vi "_Clear Capabilities.vi"(8 "error in (no error)":errorcluster, 11 "NodeDiscovery in":refnum<class "DiscoveryService.lvclass">) -> (0 "error out":errorcluster, 3 "NodeDiscovery out":refnum<class "DiscoveryService.lvclass">)   [LabVIEW 2020, in "Vecto.lvlib" / "DiscoveryService.lvclass"]
uses:
  DiscoveryService.lvclass
  DiscoveryService.lvclass/DiscoveryService.ctl
  Node Config/Node Config.lvclass
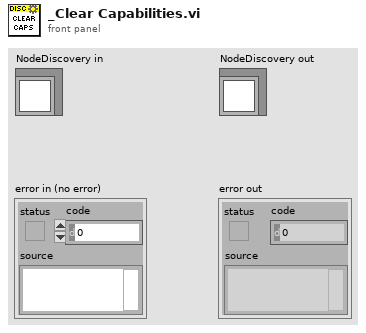
[diagram p1: front panel]
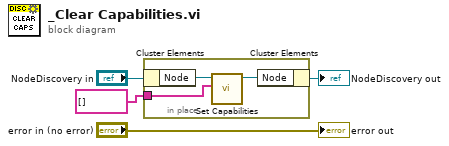
[diagram p0: block diagram]
diagram:
  n1 = in-place {
    in-place-border: string[] [] ("Capabilities") -> [w6]
    n2 = in-place-cluster #1("NodeDiscovery in") -> ("Node"=w7:refnum<class "Node Config.lvclass">)
    n3 = call "Set Capabilities.vi"("Capabilities"=w6, "Node Config in"=w7) -> ("Node Config out"=w5:refnum<class "Node Config.lvclass">)  [unwired: 8 in, 1 out]
    n4 = in-place-cluster #1("Node"=w5) -> (→"NodeDiscovery out":refnum<class "DiscoveryService.lvclass">)
  }
  "error out" <- "error in (no error)"
